vi "Read Drive Config.vi"(8 "error in (no error)":errorcluster, 10 "Drive Config Element":refnum<class "Config Element.lvclass">) -> (0 "error out":errorcluster, 2 "Drive Config":T1)   [LabVIEW 2020, in "Volatus.lvlib" / "System Health Module.lvclass"]
uses:
  System Health Module.lvclass
  System Health Module.lvclass/System Health Module.ctl
  lv-cdm/CDM-Config/Config Element/Config Element.lvclass
  Drive Config.ctl
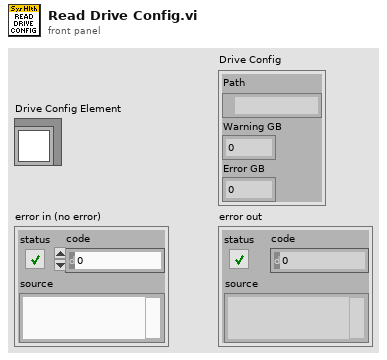
[diagram p1: front panel]
types:
  T1 = typedef "Volatus.lvlib/System Health Module.lvclass/Drive Config.ctl" = cluster{"Path":path, "Warning GB":dbl, "Error GB":dbl}
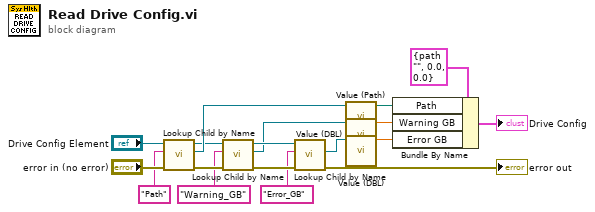
[diagram p0: block diagram]
diagram:
  n1 = call "Lookup Child by Name.vi"("error in (no error)"="error in (no error)", "Name"="Path", "Config Element in"="Drive Config Element") -> ("error out"=w14:errorcluster, "Child"=w18:refnum<class "Config Element.lvclass">, "Config Element out"=w15:refnum<class "Config Element.lvclass">)  [unwired: 5 in, 1 out]
  n2 = call "Lookup Child by Name.vi"("error in (no error)"=w14, "Name"="Warning_GB", "Config Element in"=w15) -> ("error out"=w12:errorcluster, "Child"=w8:refnum<class "Config Element.lvclass">, "Config Element out"=w13:refnum<class "Config Element.lvclass">)  [unwired: 5 in, 1 out]
  n3 = call "Lookup Child by Name.vi"("error in (no error)"=w12, "Name"="Error_GB", "Config Element in"=w13) -> ("error out"=→"error out":errorcluster, "Child"=w7:refnum<class "Config Element.lvclass">)  [unwired: 5 in, 2 out]
  n4 = call "Value (Path).vi"("Config Element in"=w18) -> ("Path Value"=w5:path)  [unwired: 9 in, 1 out]
  n5 = call "Value (DBL).vi"("Config Element in"=w8) -> ("DBL Value"=w4:dbl)  [unwired: 9 in, 1 out]
  n6 = call "Value (DBL).vi"("Config Element in"=w7) -> ("DBL Value"=w3:dbl)  [unwired: 9 in, 1 out]
  n7 = Bundle By Name(cluster=T1 {"Path"=path "", "Warning GB"=0.0, "Error GB"=0.0} ("Drive Config"), "Path"=w5, "Warning GB"=w4, "Error GB"=w3) -> (→"Drive Config":T1)
